vi "sick 624 h drive code.vi"   [LabVIEW 2016]
uses:
  Robot Global Data.vi
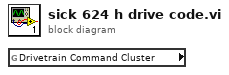
[diagram p0: block diagram]
diagram:
  n1 = global read "Robot Global Data.vi" "Drivetrain Command Cluster"() -> ()  [unwired: 1 out]
